vi "myQuake Communicate.vi"(5 "samples per chan (125)":i32=125, 6 "accelerometer settings":T1(array[cluster])=[{"Direction"=enum."Off", "Sensitivity"=FALSE}, {"Direction"=enum."Off", "Sensitivity"=FALSE}], 8 "error in (no error)":errorcluster, 9 "set offset (F)":bool, 10 "motor output (0%)":dbl(slide) scale=0.0..100.0, 11 "task array In":refnum<k21>[](array[refnum])) -> (0 "error out":errorcluster, 2 "accel data (g)":waveform(dbl)[](array[waveform]), 3 "task array out":refnum<k21>[](array[refnum]))   [LabVIEW 2013]
doc: "Writes myQuake multiplexor settings when they are updated.\n\nWrite the a PWM signal to AO0 to control the drive motor by using the <b>motor outputs</b> input.\n\nReads accelerometer data from both analog input channels.\nThe <b> set offset</b> input will store the current DC offset and subtract it from the signal."
uses:
  <vilib>/DAQmx/write.llb/DAQmx Write (Digital 1D Bool NChan 1Samp 1Line).vi
  <vilib>/DAQmx/read.llb/DAQmx Read (Analog 1D Wfm NChan NSamp).vi
  <vilib>/Analysis/baseanly.llb/Mean (DBL).vi
  <vilib>/DAQmx/miscellaneous.llb/DAQmx Fill In Error Info.vi
  <vilib>/measure/mascope.llb/Amplitude and Levels 1 chan.vi
  <vilib>/measure/NI_MAPro.lvlib
  <vilib>/Analysis/NI_AALBase.lvlib
panel:
  out "metaData":cluster{"offsets (V)":dbl[], "Y max (g)":dbl[]}
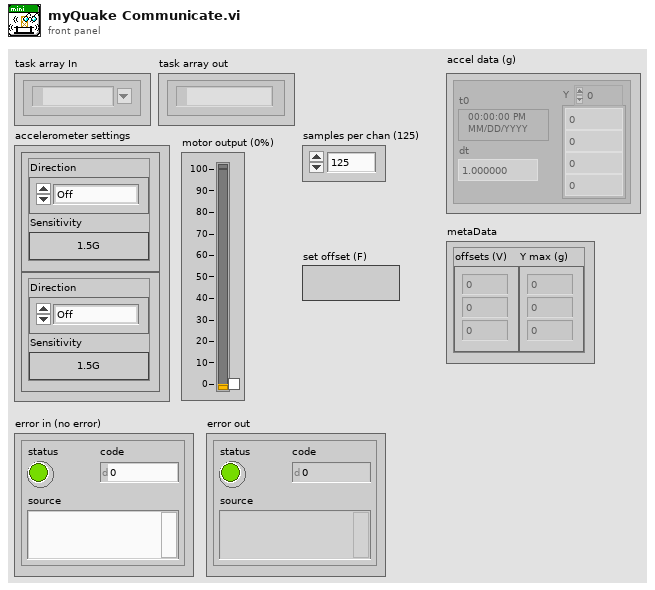
[diagram p1: front panel]
types:
  T1 = cluster{"Direction":enum16{"Off", "X - Direction", "Y - Direction", "Z - Direction"}, "Sensitivity":bool}[]
  T2 = cluster{"Direction":enum16{"Off", "X - Direction", "Y - Direction", "Z - Direction"}, "Sensitivity":bool}
  T3 = enum16{"Off", "X - Direction", "Y - Direction", "Z - Direction"}
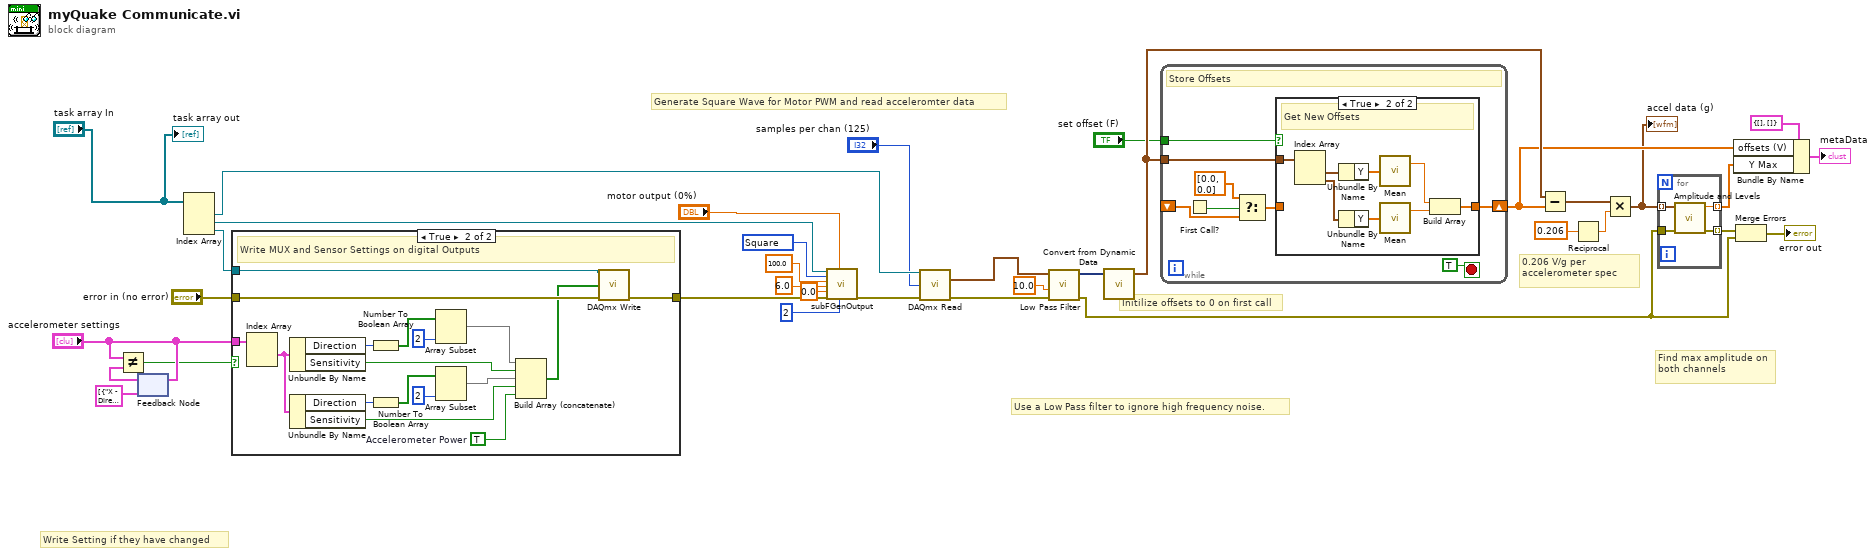
[diagram p0: block diagram]
diagram:
  w6 = 14753 items=["Sine"=14751, "Triangle"=14752, "Square"=14753, "Sawtooth"=14754] ("AO.FuncGen.Type")
  # "Generate Square Wave for Motor PWM and read acceleromter data"
  # "Find max amplitude on both channels"
  # "Use a Low Pass filter to ignore high frequency noise."
  # "Initilize offsets to 0 on first call"
  # "Write Setting if they have changed"
  # "0.206 V/g per accelerometer spec"
  n1 = feedback-in #1("accelerometer settings") -> ()
  n2 = feedback #1(T1 [{"Direction"=enum."X - Direction", "Sensitivity"=FALSE}, {"Direction"=enum."X - Direction", "Sensitivity"=FALSE}] ("Acell Settings")) -> (w27:T1)
  n3 = Not Equal?(x="accelerometer settings", y=w27) -> (x != y?=w8:bool)
  n4 = Index Array(array="task array In") -> (element #1=w29:refnum<k21>, element #2=w28:refnum<k21>, element #3=w30:refnum<k21>)  [unwired: 3 in]
  n5 = case "Write MUX settings (Dig)" shown="True" w8 {
    tunnel: "accelerometer settings" -> [_ w50]
    tunnel: w30 -> [_ w40]
    tunnel: "error in (no error)" -> [w36 w38]
    tunnel: [w36 w39] -> w35
    frame False {
      # "No change is settings, do not update digital lines"
    }
    frame True {
      w53 = TRUE  # Accelerometer Power
      # "Write MUX and Sensor Settings on digital Outputs"
      n6 = Index Array(array=w50) -> (element #1=w52:T2)  [unwired: 2 in, 1 out]
      n7 = Unbundle By Name(w52) -> ("Direction"=w47:T3, "Sensitivity"=w42:bool)
      n8 = Unbundle By Name(w52) -> ("Direction"=w44:T3, "Sensitivity"=w51:bool)
      n9 = Number To Boolean Array(number=w47) -> (Boolean array=w49:bool[])
      n10 = Number To Boolean Array(number=w44) -> (Boolean array=w45:bool[])
      n11 = Array Subset(array=w49, length=2) -> (w41:bool[])  [unwired: 1 in]
      n12 = Array Subset(array=w45, length=2) -> (w43:bool[])  [unwired: 1 in]
      n13 = Build Array (concatenate)(w41, w42, w43, w51, w53) -> (w37:bool[])
      n14 = call-poly <vilib>:"DAQmx Write.vi"("task/channels in"=w40, "data"=w37, "error in"=w38) -> ("error out"=w39:errorcluster)  [unwired: 10 in, 2 out]
    }
  }
  n15 = call <vilib>:"subFGenOutput.vi"("task in"=w28, "AO.FuncGen.Type"=w6, "Frequency"=100.0 ("frequency"), "Amplitude"=6.0 ("amplitude"), "Offset"=0.0, "error in (no error)"=w35, "square wave duty cycle (%)"="motor output (0%)", "Signal Type"=2) -> ("error out"=w5:errorcluster)  [unwired: 9 in, 2 out]
  n16 = call-poly <vilib>:"DAQmx Read.vi"("task/channels in"=w29, "number of samples per channel"="samples per chan (125)", "error in"=w5) -> ("data"=w25:waveform(dbl)[], "error out"=w31:errorcluster)  [unwired: 10 in, 1 out]
  n17 = call "Low Pass Filter"("error in (no error)"=w31, "Lower Cut-Off"=10.0, "Signal"=w25) -> ("error out"=w9:errorcluster, "Filtered Signal"=w34:dynamicdata)  [unwired: 7 in]
  n18 = call "Convert from Dynamic Data"("Dynamic Data Type"=w34) -> ("Array of Waveform"=w21:waveform(dbl)[])  [unwired: 3 in]
  n19 = while "Store Offsets" {
    tunnel: w21 -> [w61]
    shift-right: [w60] -> w20
    shift-left: _ -> [w55]
    tunnel: "set offset (F)" -> [w58]
    stop <- TRUE stop-if-true
    # "Store Offsets"
    n20 = First Call?() -> (First Call?: T/F=w57:bool)
    n21 = Select(t=dbl[] [0.0, 0.0], s=w57, f=w55) -> (s? t:f=w54:dbl[])
    n22 = case shown="True" w58 {
      tunnel: w61 -> [_ w66]
      tunnel: [w62 w63] -> w60
      tunnel: w54 -> [w62 _]
      frame False {
        # "Use existing Offsets"
      }
      frame True {
        # "Get New Offsets"
        n23 = Index Array(array=w66) -> (element #1=w68:waveform(dbl), element #2=w67:waveform(dbl))  [unwired: 2 in]
        n24 = Unbundle By Name(w68) -> ("Y"=w65:dbl[])
        n25 = Unbundle By Name(w67) -> ("Y"=w64:dbl[])
        n26 = call-poly <vilib>:"Mean.vi"("X"=w65) -> ("mean"=w70:dbl)  [unwired: 1 out]
        n27 = call-poly <vilib>:"Mean.vi"("X"=w64) -> ("mean"=w69:dbl)  [unwired: 1 out]
        n28 = Build Array(w70, w69) -> (w63:dbl[])
      }
    }
  }
  n29 = Subtract(x=w21, y=w20) -> (x-y=w19:waveform(dbl)[])
  n30 = Reciprocal(x=0.206) -> (1/x=w32:dbl)
  n31 = Multiply(x=w19, y=w32) -> (x*y=w11:waveform(dbl)[])
  "accel data (g)" <- w11
  n32 = for {
    tunnel: w11 -> [w74] mode=indexing
    tunnel: [w73] -> w23 mode=indexing
    tunnel: w9 -> [w72]
    tunnel: [w71] -> w22 mode=indexing
    n33 = call-poly <vilib>:"Amplitude and Levels.vi"("error in (no error)"=w72, "signal in"=w74) -> ("error out"=w71:errorcluster, "amplitude"=w73:dbl)  [unwired: 6 in, 2 out]
  }
  n34 = Bundle By Name(cluster=cluster{"offsets (V)":dbl[], "Y Max":dbl[]} {"offsets (V)"=[], "Y Max"=[]}, "offsets (V)"=w20, "Y Max"=w23) -> (→"metaData":cluster{"offsets (V)":dbl[], "Y Max":dbl[]})
  n35 = Merge Errors(w22, w9) -> (→"error out":errorcluster)
  "task array out" <- "task array In"
